vi "arun2.vi"() -> ()   [LabVIEW 2020]
panel:
  out "Array":string[](array[string])
  out "size(s)":i32[](array[numeric])
  out "output array":i32[][](array[numeric])
  out "element 2":i32
  out "element":i32
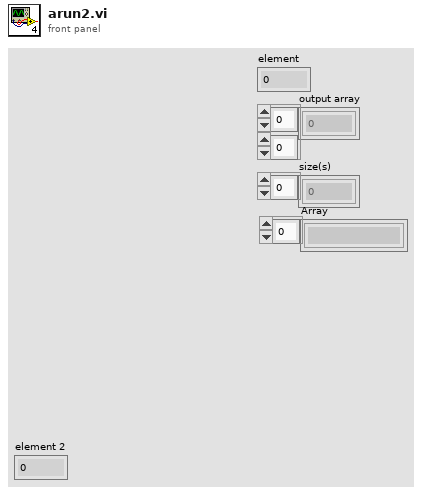
[diagram p1: front panel]
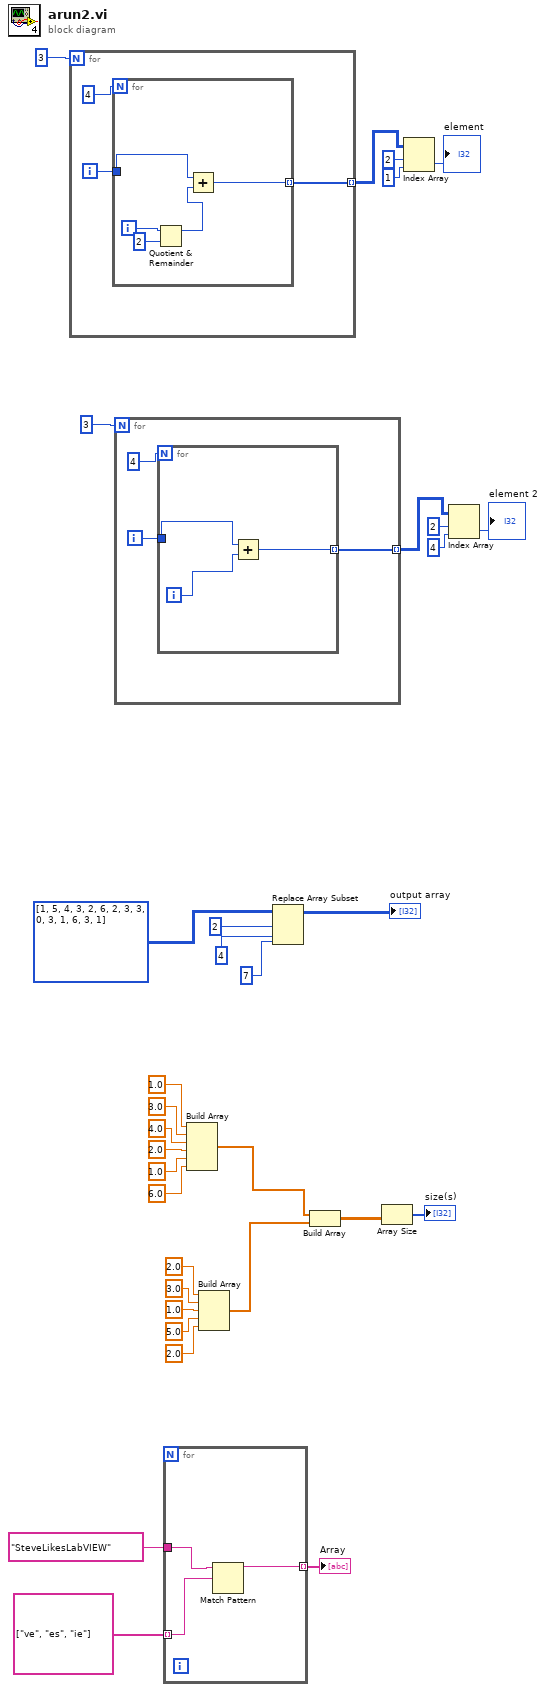
[diagram p0: block diagram]
diagram:
  n1 = for {
    N: 3 -> [_]
    tunnel: [w34] -> w32 mode=indexing
    i -> [w35]
    n2 = for {
      N: 4 -> [_]
      tunnel: w35 -> [w41]
      tunnel: [w40] -> w34 mode=indexing
      i -> [w39]
      n3 = Quotient & Remainder(x=w39, y=2) -> (x-y*floor(x/y)=w37:i32)  [unwired: 1 out]
      n4 = Add(x=w41, y=w37) -> (x+y=w40:i32)
    }
  }
  n5 = for {
    N: 3 -> [_]
    tunnel: [w42] -> w27 mode=indexing
    i -> [w43]
    n6 = for {
      N: 4 -> [_]
      tunnel: w43 -> [w47]
      tunnel: [w46] -> w42 mode=indexing
      i -> [w45]
      n7 = Add(x=w47, y=w45) -> (x+y=w46:i32)
    }
  }
  n8 = for {
    tunnel: "SteveLikesLabVIEW" -> [w50]
    tunnel: string[] ["ve", "es", "ie"] -> [w49] mode=indexing
    tunnel: [w48] -> w1 mode=indexing
    n9 = Match Pattern(string=w50, regular expression=w49) -> (before substring=w48:string)  [unwired: 1 in, 3 out]
  }
  "Array" <- w1
  n10 = Build Array(1.0 ("element"), 3.0 ("element"), 4.0 ("element"), 2.0 ("element"), 1.0 ("element"), 6.0 ("element")) -> (w7:dbl[])
  n11 = Build Array(2.0 ("element"), 3.0 ("element"), 1.0 ("element"), 5.0 ("element"), 2.0 ("element")) -> (w6:dbl[])
  n12 = Replace Array Subset "Replace Array Subset"(array=i32[][] [[1, 5, 4, 3, 2], [6, 2, 3, 3, 0], [3, 1, 6, 3, 1]], new element=7, index (row)=2, index (col)=4) -> (→"output array":i32[][])
  n13 = Build Array(w7, w6) -> (w5:dbl[][])
  n14 = Array Size(array=w5) -> (size(s)=→"size(s)":i32[])
  n15 = Index Array(array=w32, index (row)=2, index (col)=1 ("disabled index (col)")) -> (element=→"element":i32)
  n16 = Index Array "Index Array"(array=w27, index (row)=2, index (col)=4 ("disabled index (col)")) -> (element=→"element 2":i32)
